vi "Labview1.vi"() -> ()   [LabVIEW 2015]
panel:
  in  "milliseconds to wait":u32
  in  "stop":bool
  in  "Temperature (F)":dbl(slide) scale=0.0..200.0
  out "Thermometer (C)":dbl(slide) scale=0.0..100.0
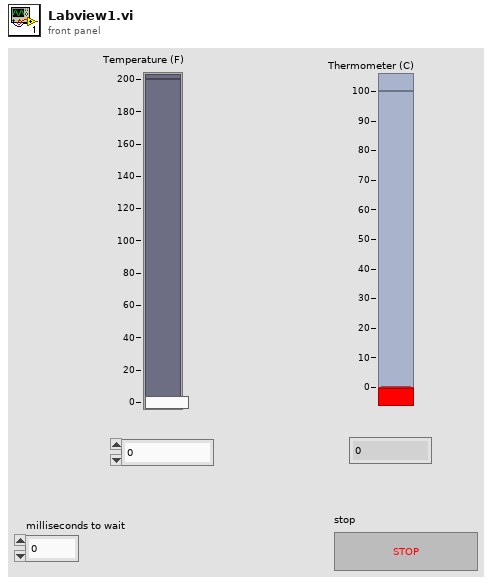
[diagram p1: front panel]
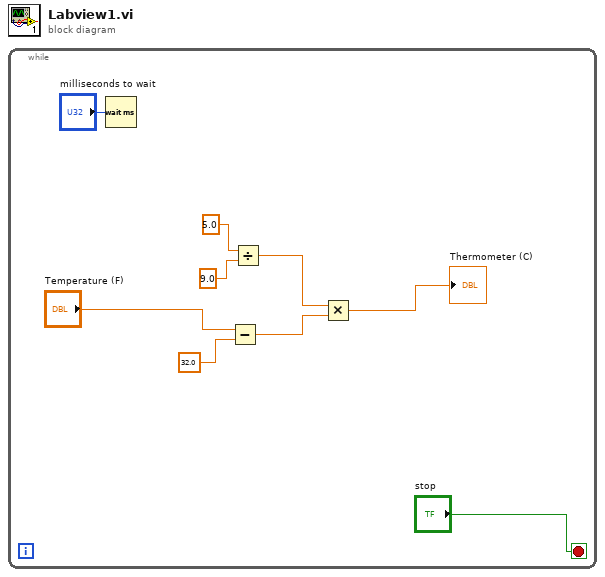
[diagram p0: block diagram]
diagram:
  n1 = while {
    stop <- "stop" stop-if-true
    n2 = Wait (ms)(milliseconds to wait="milliseconds to wait") -> ()  [unwired: 1 out]
    n3 = Subtract(x="Temperature (F)", y=32.0) -> (x-y=w8:dbl)
    n4 = Divide(x=5.0, y=9.0) -> (x/y=w7:dbl)
    n5 = Multiply(x=w7, y=w8) -> (x*y=→"Thermometer (C)":dbl)
  }
